vi "Phasor Compute Gate-IRF Array.vi"(8 "Error In":errorcluster, 9 "Gate & Decay Parameters":T1 {"A" format="%#_4g"; "s" format="%#_4g"; "sF" format="%#_4g"; "sR" format="%#_4g"; "t_i" format="%#_4g"; "t_0" format="%#_4g"; "tau" format="%#_4g"; "T" format="%#_4g"; "W" format="%#_4g"}, 11 "X":dbl[](array[numeric])) -> (0 "Error Out":errorcluster, 3 "IRF/Gate Array":dbl[](array[numeric]))   [LabVIEW 2021, in "Phasor.lvlib"]
uses:
  Phasor.lvlib
  Phasor Gate & Decay Parameters.ctl
  Phasor Gate Type.ctl
  Phasor IRF Model.ctl
  Graphs/XY Graph/XY Graph Plot Data.ctl
  7d9bb666-8e44-4efd-bf11-38a816117c5c.vi
  <vilib>/Utility/error.llb/Error Cluster From Error Code.vi
  Math/Math.lvlib
  Graphs/XY Graph/XY Graph Add-Ons.lvlib
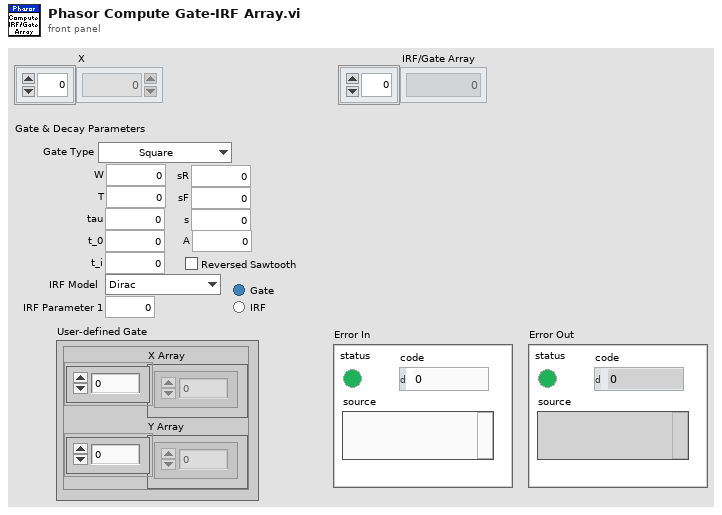
[diagram p1: front panel]
types:
  T1 = typedef "Phasor.lvlib/Phasor Gate & Decay Parameters.ctl" = cluster{"W":dbl, "T":dbl, "tau":dbl, "t_0":dbl, "Gate Type":T2, "t_i":dbl, "sR":dbl, "sF":dbl, "s":dbl, "Reversed Sawtooth":bool, "IRF Model":T3, "IRF Parameter 1":dbl, "User-defined Gate":T4, "Type of User-defined Function":enum32{"Gate", "IRF"}, "A":dbl}
  T2 = typedef "Phasor.lvlib/Phasor Gate Type.ctl" = enum16{"Square", "Finite Edge Square", "Finite Edge, Tilted Top Square", "Triangle", "Sawtooth", "User-defined"}
  T3 = typedef "Phasor.lvlib/Phasor IRF Model.ctl" = enum16{"Dirac", "Exponential"}
  T4 = typedef "XY Graph Add-Ons.lvlib/XY Graph Plot Data.ctl" = cluster{"X Array":dbl[], "Y Array":dbl[]}
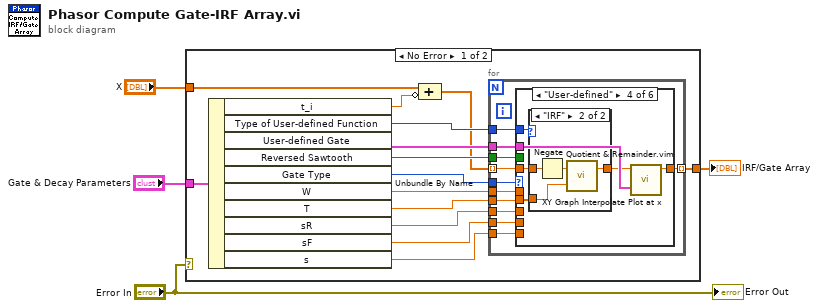
[diagram p0: block diagram]
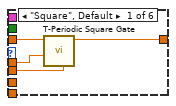
[diagram p2: hidden frame]
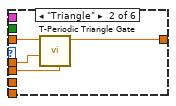
[diagram p3: hidden frame]
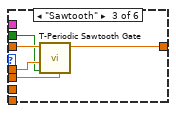
[diagram p4: hidden frame]
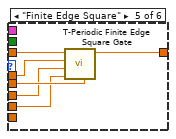
[diagram p6: hidden frame]
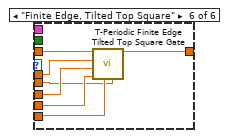
[diagram p7: hidden frame]
diagram:
  n1 = case shown="No Error" "Error In" {
    tunnel: "X" -> [w18 _]
    tunnel: "Gate & Decay Parameters" -> [w17 _]
    tunnel: [w16 _] -> w2
    frame No Error {
      n2 = Unbundle By Name(w17) -> ("t_i"=w5:dbl, "Type of User-defined Function"=w13:enum32{"Gate", "IRF"}, "User-defined Gate"=w14:T4, "Reversed Sawtooth"=w15:bool, "Gate Type"=w6:T2, "W"=w7:dbl, "T"=w8:dbl, "sR"=w11:dbl, "sF"=w10:dbl, "s"=w9:dbl)
      n3 = Compound Arithmetic op=ADD(w18, invert w5) -> (w12:dbl[])
      n4 = for {
        tunnel: w8 -> [w20]
        tunnel: w12 -> [w29] mode=indexing
        tunnel: w6 -> [w28]
        tunnel: [w27] -> w16 mode=indexing
        tunnel: w7 -> [w26]
        tunnel: w11 -> [w25]
        tunnel: w10 -> [w24]
        tunnel: w9 -> [w23]
        tunnel: w15 -> [w22]
        tunnel: w14 -> [w21]
        tunnel: w13 -> [w19]
        n5 = case shown="\"User-defined\"" w28 {
          tunnel: w26 -> [w32 w37 w41 _ w57 w64]
          tunnel: w29 -> [w33 w36 w42 w48 w59 w66]
          tunnel: [w31 w35 w40 w47 w58 w65] -> w27
          tunnel: w25 -> [_ _ _ _ w55 w63]
          tunnel: w24 -> [_ _ _ _ w54 w62]
          tunnel: w23 -> [_ _ _ _ _ w61]
          tunnel: w22 -> [_ _ w39 _ _ _]
          tunnel: w21 -> [_ _ _ w46 _ _]
          tunnel: w20 -> [w30 w34 w38 w45 w56 w60]
          tunnel: w19 -> [_ _ _ w43 _ _]
          frame "Square", Default {
            n6 = call "T-Periodic Square Gate.vi"("Period T"=w30, "W"=w32, "t"=w33) -> ("Square(t)"=w31:dbl)  [unwired: 8 in]
          }
          frame "Triangle" {
            n7 = call "T-Periodic Triangle Gate.vi"("Period T"=w34, "W"=w37, "t"=w36) -> ("Triangle(t)"=w35:dbl)  [unwired: 8 in]
          }
          frame "Sawtooth" {
            n8 = call "T-Periodic Sawtooth Gate.vi"("Period T"=w38, "Reversed?"=w39, "W"=w41, "t"=w42) -> ("Sawtooth(t)"=w40:dbl)  [unwired: 7 in]
          }
          frame "User-defined" {
            n9 = case shown="\"IRF\"" w43 {
              tunnel: w48 -> [w49 w53]
              tunnel: w45 -> [_ w51]
              tunnel: [w49 w50] -> w44
              frame "Gate", Default {
              }
              frame "IRF" {
                n10 = Negate(x=w53) -> (-x=w52:dbl)
                n11 = call "Quotient & Remainder.vim"("y"=w51, "x"=w52) -> ("x - E(x/y)y"=w50:dbl)  [unwired: 1 out]
              }
            }
            n12 = call "XY Graph Interpolate Plot at x.vi"("XY Plot"=w46, "t"=w44) -> ("XY Plot(t)"=w47:dbl)  [unwired: 8 in, 1 out]
          }
          frame "Finite Edge Square" {
            n13 = call "T-Periodic Finite Edge Square Gate.vi"("Period T"=w56, "s_F"=w54, "s_R"=w55, "W"=w57, "t"=w59) -> ("Finite Edge Square(t)"=w58:dbl)  [unwired: 6 in]
          }
          frame "Finite Edge, Tilted Top Square" {
            n14 = call "T-Periodic Finite Edge Tilted Top Square Gate.vi"("Period T"=w60, "slope"=w61, "s_F"=w62, "s_R"=w63, "W"=w64, "t"=w66) -> ("Finite Edge Square(t)"=w65:dbl)  [unwired: 5 in]
          }
        }
      }
    }
    frame Error {
    }
  }
  "IRF/Gate Array" <- w2
  "Error Out" <- "Error In"
